vi "IV-Curve.vi"() -> ()   [LabVIEW 2024]
uses:
  <vilib>/Utility/file.llb/Write Delimited Spreadsheet (DBL).vi
  <instrlib>/Keithley 648X Series/Keithley 648X Series.lvlib
panel:
  in  "Number repititions":i32=1
  in  "Filename":string="test"
  out "appended path":path=path "C:/Data/SiPM/20240318_test.h5"
  in  "Measurement Time (6 PLC)":dbl=6.0
  out "Numeric":i32
  in  "Difficulty Class":enum32{"Easy", "Medium"}(tab)
  in  "Arm Loop Count":i32=1
  in  "Arm Source":u16(ring) items=["Immediate", "Timer", "Bus", "Tlink", "Manual", "Negative SOT", "Positive SOT", "Bidirectional SOT"]
  in  "Arm Timer Interval":dbl=0.1
  in  "Enable Arm Bypass":bool
  in  "Enable Trigger Bypass":bool
  in  "Trigger Delay":dbl
  in  "Trigger Loop Count":i32=1
  in  "Trigger Source":u16(ring) items=["Immediate", "Tlink"]
  in  "Voltage Sweep Step Size":dbl=0.5
  in  "Voltage Sweep Stop":dbl=1.5
  in  "Voltage Sweep Start":dbl
  in  "Voltage Sweep Delay":dbl=1.0
  out "Voltage Sweep Results":cluster{dbl[], dbl[]}(graph)
  in  "Serial Configuration":T1={"Baud Rate"=9600, "Parity"=0, "Data Bits"=8, "Stop Bits"=10, "Flow Control"=0} {"Flow Control" items=["None", "XON/XOFF", "RTS/CTS", "XON/XOFF & RTS/CTS", "DTR/DSR", "XON/XOFF & DTR/DSR"]; "Stop Bits" items=["1.0"=10, "1.5"=15, "2.0"=20]; "Data Bits" items=["7"=7, "8"=8]; "Parity" items=["None", "Odd", "Even", "Mark", "Space"]; "Baud Rate" items=["300"=300, "600"=600, "1200"=1200, "2400"=2400, "4800"=4800, "9600"=9600, "19200"=19200]}
  in  "VISA resource name":refnum<visa-resource-name>="COM4"
  # "Configure the Sweep Settings, and the Serial Configuration if need be. Then hit the run button."
  # "Make sure that the instrument is triggered for each of the voltage measurements in the sweep. Otherwise the sweep won't execute, or it executes, but the instrument does not function as expected."
  # "Also Make sure to configure the arm and trigger layers appropriately. The Read Sweep Results relies on\na wait loop that may never terminate if the configuration is not conducive to its termination."
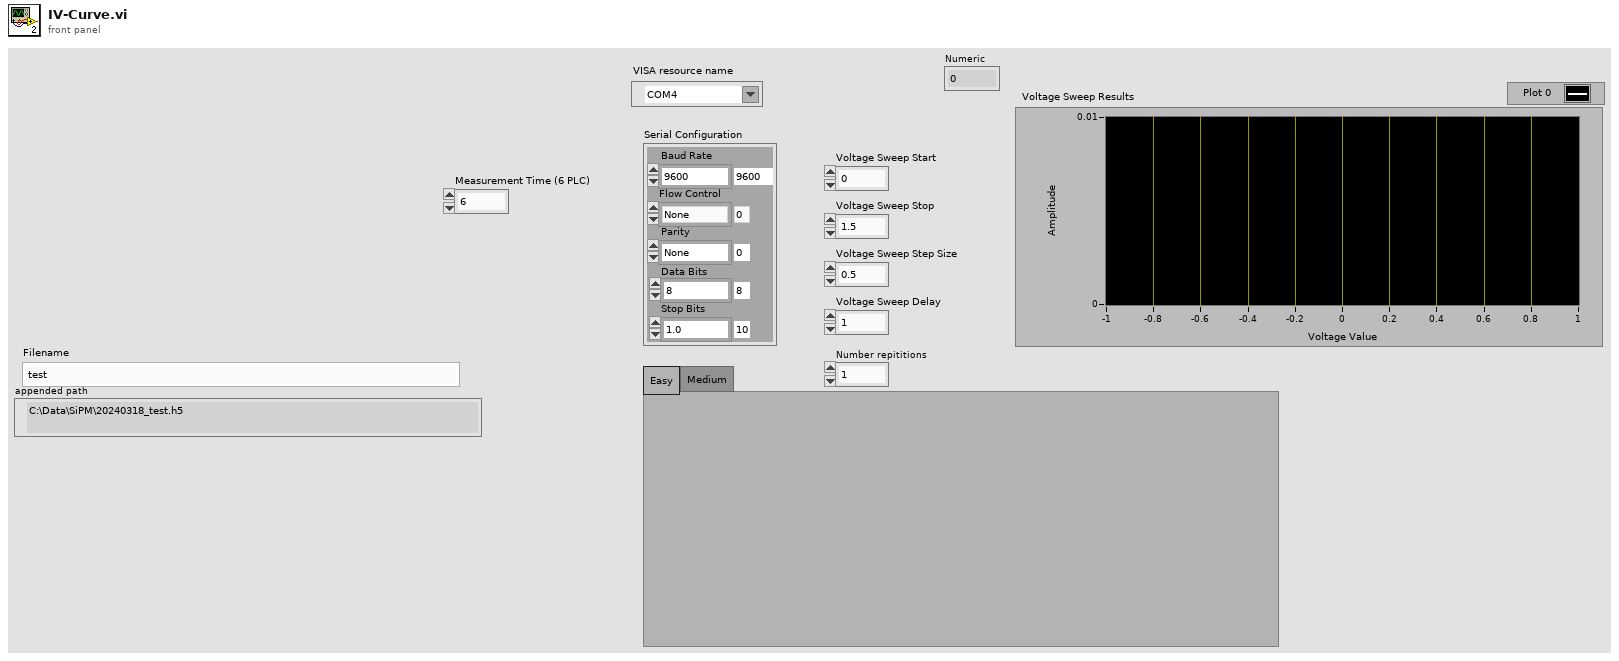
[diagram p1: front panel]
types:
  T1 = cluster{"Baud Rate":u32, "Parity":u16, "Data Bits":u16, "Stop Bits":u16, "Flow Control":u16}
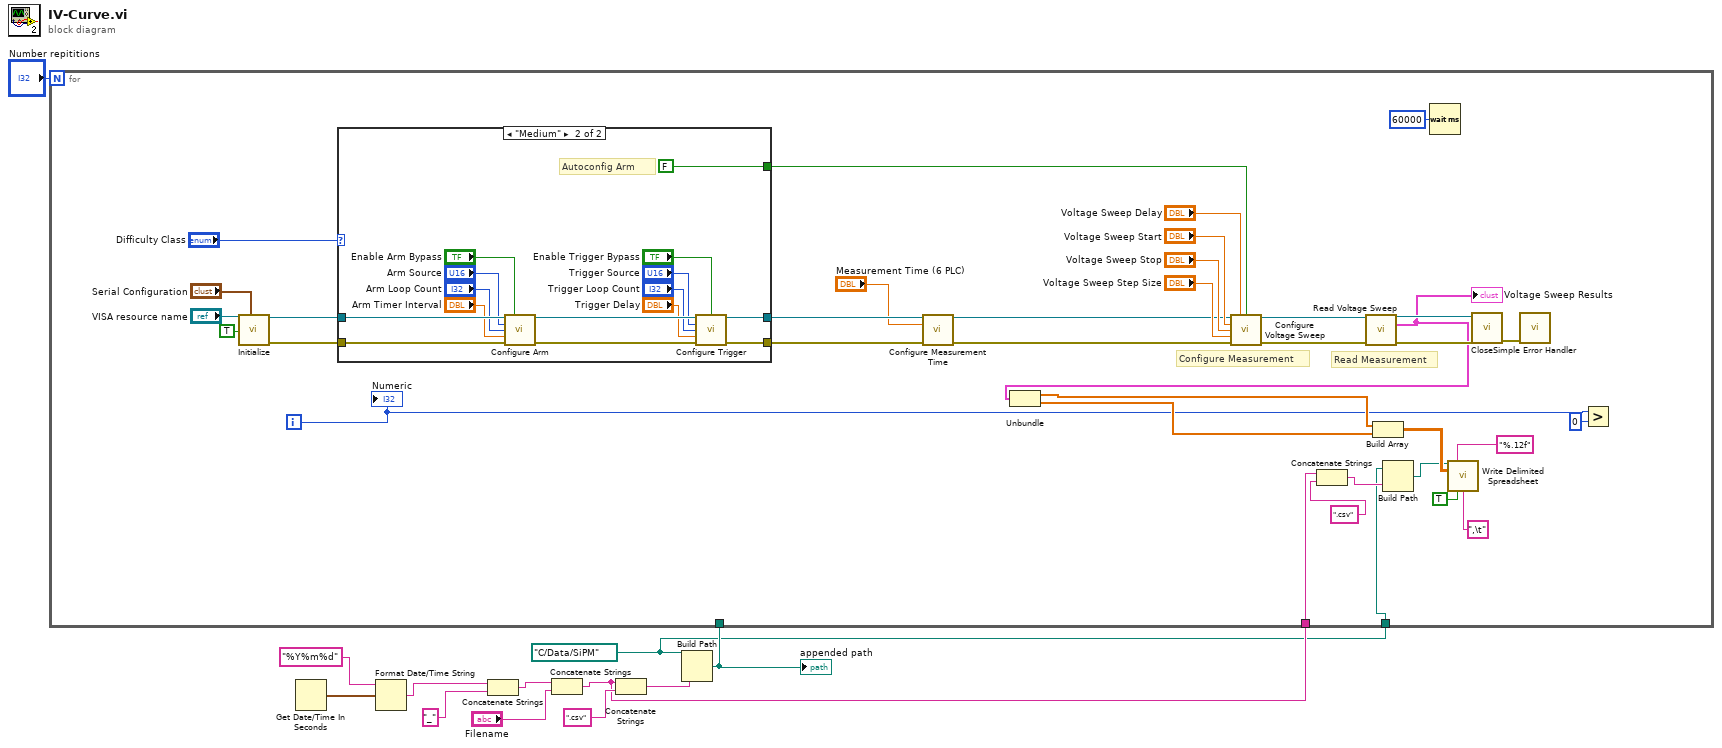
[diagram p0: block diagram]
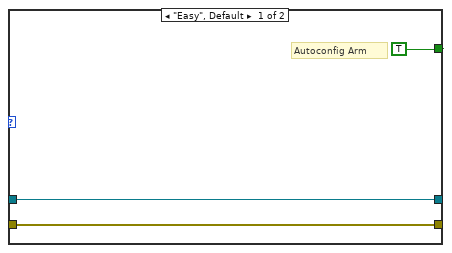
[diagram p2: hidden frame]
diagram:
  w2 = path "C:/Data/SiPM" ("base path")
  n1 = Get Date/Time In Seconds() -> (seconds since 1Jan1904=w12:timestamp)
  n2 = Format Date/Time String(time format string (%c)="%Y%m%d", seconds (now)=w12) -> (date/time string=w7:string)  [unwired: 1 in]
  n3 = Concatenate Strings(w7, "_" ("string")) -> (w5:string)
  n4 = Concatenate Strings(w5, "Filename") -> (w3:string)
  n5 = Concatenate Strings(w3, ".csv" ("string")) -> (w11:string)
  n6 = Build Path(base path=w2, name or relative path=w11) -> (appended path=w4:path)
  "appended path" <- w4
  n7 = for {
    N: "Number repititions" -> [_]
    tunnel: w4 -> [_]
    tunnel: w3 -> [w22]
    tunnel: w2 -> [w13]
    i -> [w18]
    # "Read Measurement"
    # "Configure Measurement"
    n8 = call <instrlib>:"Initialize.vi"("Serial Configuration"="Serial Configuration", "ID Query (True)"=TRUE, "VISA resource name"="VISA resource name") -> ("error out"=w36:errorcluster, "VISA resource name out"=w37:refnum<visa-resource-name>)  [unwired: 7 in]
    n9 = case shown="\"Medium\"" "Difficulty Class" {
      tunnel: [w51 w60] -> w32
      tunnel: w37 -> [w51 w65]
      tunnel: w36 -> [w50 w64]
      tunnel: [w50 w62] -> w30
      tunnel: [TRUE FALSE] -> w34
      frame "Easy", Default {
        # "Autoconfig Arm"
      }
      frame "Medium" {
        # "Autoconfig Arm"
        n10 = call <instrlib>:"Configure Arm.vi"("VISA resource name"=w65, "Enable Arm Bypass (F: Disable)"="Enable Arm Bypass", "Arm Source (0: Immediate)"="Arm Source", "Arm Loop Count (1)"="Arm Loop Count", "Arm Timer Interval (0.1 s)"="Arm Timer Interval", "error in (no error)"=w64) -> ("VISA resource name out"=w61:refnum<visa-resource-name>, "error out"=w63:errorcluster)  [unwired: 8 in]
        n11 = call <instrlib>:"Configure Trigger.vi"("VISA resource name"=w61, "Enable Trigger Bypass (F: Disable)"="Enable Trigger Bypass", "Trigger Source (0: Immediate)"="Trigger Source", "Trigger Loop Count (1)"="Trigger Loop Count", "Trigger Delay (0 s)"="Trigger Delay", "error in (no error)"=w63) -> ("VISA resource name out"=w60:refnum<visa-resource-name>, "error out"=w62:errorcluster)  [unwired: 8 in]
      }
    }
    n12 = call <instrlib>:"Configure Measurement Time.vi"("VISA resource name"=w32, "Measurement Time (6 PLC)"="Measurement Time (6 PLC)", "error in (no error)"=w30) -> ("VISA resource name out"=w31:refnum<visa-resource-name>, "error out"=w29:errorcluster)  [unwired: 11 in]
    n13 = call <instrlib>:"Configure Voltage Sweep.vi"("VISA resource name"=w31, "Voltage Sweep Delay (1s)"="Voltage Sweep Delay", "Autoconfig Arm (T: Enable)"=w34, "Voltage Sweep Start (0V)"="Voltage Sweep Start", "Voltage Sweep Stop (10V)"="Voltage Sweep Stop", "Voltage Sweep Step Size (1V)"="Voltage Sweep Step Size", "error in (no error)"=w29) -> ("VISA resource name out"=w43:refnum<visa-resource-name>, "error out"=w42:errorcluster)  [unwired: 7 in]
    n14 = Concatenate Strings(w22, ".csv") -> (w19:string)
    n15 = call <instrlib>:"Read Voltage Sweep.vi"("VISA resource name"=w43, "error in (no error)"=w42) -> ("VISA resource name out"=w44:refnum<visa-resource-name>, "Voltage Sweep Results"=w26:cluster{dbl[], dbl[]}, "error out"=w45:errorcluster)  [unwired: 11 in]
    "Voltage Sweep Results" <- w26
    n16 = Unbundle(w26) -> (w25:dbl[], w24:dbl[])
    n17 = Build Array(w25, w24) -> (w23:dbl[][])
    n18 = Build Path(base path=w13, name or relative path=w19) -> (appended path=w20:path)
    n19 = Wait (ms)(milliseconds to wait=u32 60000) -> ()  [unwired: 1 out]
    n20 = call-poly <vilib>:"Write Delimited Spreadsheet.vi"("file path (dialog if empty)"=w20, "format (%.3f)"="%.12f", "2D data"=w23, "transpose? (no:F)"=TRUE, "delimiter (\\t)"=",\t" ("delimiter (\\t)")) -> ()  [unwired: 9 in, 2 out]
    n21 = call <instrlib>:"Close.vi"("error in (no error)"=w45, "VISA resource name"=w44) -> ("error out"=w48:errorcluster)  [unwired: 9 in]
    n22 = call <vilib>:"Simple Error Handler.vi"("error in (no error)"=w48) -> ()  [unwired: 4 in, 5 out]
    n23 = Greater?(x=w18, y=0) -> ()  [unwired: 1 out]
    "Numeric" <- w18
  }
